vi "THzTime_SPEED_control_reduced.vi"(1 "ESP300 Axis":i8=1, 2 "ESP300 Address":string="1", 4 "Lockin Address":string="12") -> ()   [LabVIEW 2010]
panel:
  in  "Axis Number":u8
  in  "SHOT202 Address":string
  in  "reference postion":dbl
  in  "sample position":dbl
  in  "number of measurement":dbl
  in  "Interdelay (ms)":dbl
  in  "pre delay(ms)":dbl=10.0
  in  "Reset Range":bool
  out "Lock-in Y-Channel":dbl=2.5466e-11 format="%#.3p"
  out "Lock-in X-Channel":dbl=-5.457e-12 format="%#.3p"
  out "THz Time-domain Signal Wave":cluster{"x-axis":sgl[], "y-axis":dbl[]}(graph)={"x-axis"=[-3.0, -2.99, -2.98, -2.97, -2.96, -2.95, -2.94, -2.93, -2.92, -2.91, -2.9, -2.89, -2.88, -2.87, -2.86, -2.85, -2.84, -2.83, -2.82, -2.81, -2.8, -2.79, -2.78, -2.77, -2.76, -2.75, -2.74, -2.73, -2.72, -2.71, -2.7, -2.69, -2.68, -2.67, -2.66, -2.65, -2.64, -2.63, -2.6200001, -2.61, -2.6, -2.59, -2.58, -2.57, -2.56, -2.55, -2.54, -2.53, -2.52, -2.51, -2.5, -2.49, -2.48, -2.47, -2.46, -2.45, -2.44, -2.43, -2.42, -2.41, -2.4, -2.39, -2.38, -2.3700001, -2.3600001, -2.35, -2.34, -2.33, -2.32, -2.31, -2.3, -2.29, -2.28, -2.27, -2.26, -2.25, -2.24, -2.23, -2.22, -2.21, -2.2, -2.19, -2.18, -2.17, -2.16, -2.15, -2.14, -2.13, -2.1200001, -2.1100001, -2.1, -2.09, -2.08, -2.07, -2.06, -2.05, -2.04, -2.03, -2.02, -2.01, -2.0, -1.99, -1.98, -1.97, -1.96, -1.95, -1.94, -1.9300001, -1.9200001, -1.91, -1.9, -1.89, -1.88, -1.87, -1.86, -1.85, -1.84, -1.83, -1.82, -1.8100001, -1.8000001, -1.7900001, -1.78, -1.77, -1.76, -1.75, -1.74, -1.73, -1.72, -1.71, -1.7, -1.69, -1.6800001, -1.6700001, -1.6600001, -1.65, -1.64, -1.63, -1.62, -1.61, -1.6, -1.59, -1.58, -1.57, -1.5600001, -1.5500001, -1.5400001, -1.5300001, -1.52, -1.51, -1.5, -1.49, -1.48, -1.47, -1.46, -1.45, -1.44, -1.4300001, -1.4200001, -1.4100001, -1.4000001, -1.39, -1.38, -1.37, -1.36, -1.35, -1.34, -1.33, -1.32, -1.3100001, -1.3000001, -1.2900001, -1.2800001, -1.27, -1.26, -1.25, -1.24, -1.23, -1.22, -1.21, -1.2, -1.19, -1.1800001, -1.1700001, -1.1600001, -1.1500001, -1.14, -1.13, -1.12, -1.11, -1.1, -1.09, -1.08, -1.07, -1.0600001, -1.0500001, -1.0400001, -1.0300001, -1.0200001, -1.01, -1.0, -0.99000007], "y-axis"=[6.18461e-11, 6.18461e-11, 6.275559999999999e-11, 6.457460000000001e-11, 6.54841e-11, 6.63936e-11, 6.821255e-11, 7.00315e-11, 7.18505e-11, 7.36695e-11, 7.54885e-11, 7.6398e-11, 7.6398e-11, 7.8217e-11, 7.8217e-11, 7.8217e-11, 7.8217e-11, 7.8217e-11, 7.8217e-11, 7.8217e-11, 7.8217e-11, 7.8217e-11, 7.8217e-11, 7.8217e-11, 7.73075e-11, 7.6398e-11, 7.54885e-11, 7.4579e-11, 7.4579e-11, 7.4579e-11, 7.4579e-11, 7.4579e-11, 7.4579e-11, 7.4579e-11, 7.36695e-11, 7.276e-11, 7.276e-11, 7.276e-11, 7.18505e-11, 7.18505e-11, 7.276e-11, 7.18505e-11, 7.0941e-11, 7.0941e-11, 7.00315e-11, 6.9122e-11, 6.821255e-11, 6.63936e-11, 6.457460000000001e-11, 6.275559999999999e-11, 6.18461e-11, 6.18461e-11, 6.275559999999999e-11, 6.36651e-11, 6.63936e-11, 6.912205e-11, 7.275999999999999e-11, 7.6398e-11, 7.91265e-11, 8.09455e-11, 8.27645e-11, 8.3674e-11, 8.3674e-11, 8.3674e-11, 8.27645e-11, 8.09455e-11, 7.821699999999999e-11, 7.36695e-11, 6.821255e-11, 6.09366e-11, 5.54795e-11, 4.911295e-11, 4.2746500000000003e-11, 3.7289500000000003e-11, 3.2742e-11, 3.001355e-11, 2.7285e-11, 2.7285e-11, 2.819455e-11, 3.092305e-11, 3.4561000000000003e-11, 3.7289500000000003e-11, 3.9108499999999995e-11, 4.09275e-11, 4.45655e-11, 4.638445e-11, 5.00224e-11, 5.18414e-11, 5.36604e-11, 5.72985e-11, 5.82081e-11, 5.82081e-11, 5.82081e-11, 6.00271e-11, 6.09366e-11, 6.275559999999999e-11, 6.457460000000001e-11, 6.730305e-11, 7.00315e-11, 7.18505e-11, 7.36695e-11, 7.54885e-11, 7.6398e-11, 7.73075e-11, 7.8217e-11, 7.8217e-11, 7.8217e-11, 7.8217e-11, 7.8217e-11, 7.8217e-11, 7.8217e-11, 7.8217e-11, 7.8217e-11, 7.8217e-11, 7.8217e-11, 7.8217e-11, 7.91265e-11, 8.0036e-11, 8.0036e-11, 7.91265e-11, 7.8217e-11, 7.8217e-11, 7.8217e-11, 7.8217e-11, 7.91265e-11, 8.0036e-11, 8.0036e-11, 8.0036e-11, 8.09455e-11, 8.1855e-11, 8.09455e-11, 8.0036e-11, 7.91265e-11, 7.8217e-11, 7.8217e-11, 7.73075e-11, 7.54885e-11, 7.36695e-11, 7.18505e-11, 6.9122e-11, 6.73031e-11, 6.54841e-11, 6.457460000000001e-11, 6.36651e-11, 6.275559999999999e-11, 6.09366e-11, 6.00271e-11, 6.00271e-11, 6.00271e-11, 6.00271e-11, 6.09366e-11, 6.18461e-11, 6.18461e-11, 6.18461e-11, 6.275559999999999e-11, 6.36651e-11, 6.457460000000001e-11, 6.54841e-11, 6.457460000000001e-11, 6.36651e-11, 6.36651e-11, 6.36651e-11, 6.36651e-11, 6.36651e-11, 6.36651e-11, 6.36651e-11, 6.36651e-11, 6.36651e-11, 6.36651e-11, 6.36651e-11, 6.36651e-11, 6.36651e-11, 6.457460000000001e-11, 6.54841e-11, 6.457460000000001e-11, 6.457460000000001e-11, 6.54841e-11, 6.63936e-11, 6.73031e-11, 6.73031e-11, 6.9122e-11, 6.73031e-11, 6.821255e-11, 6.9122e-11, 6.9122e-11, 6.73031e-11, 6.821255e-11, 6.9122e-11, 6.9122e-11, 6.9122e-11, 6.9122e-11, 6.821255e-11, 6.73031e-11, 6.73031e-11, 6.73031e-11, 6.73031e-11, 6.73031e-11, 6.73031e-11, 6.63936e-11, 6.63936e-11, 6.54841e-11, 6.54841e-11]}
  in  "Autosave Directory for Long-term Average Scan":path=path "D:/KHA/20140828_reference/20140829/MAX1"
  in  "OK Button":bool
  out "Data Type":string="outp ? 1"
  in  "Enum":enum16{"X", "Y", "Abs"}(ring)
  in  "Draw":bool
  in  "Exit Program":bool
  in  "Short term \nAverage#":i8=2
  in  "Step":sgl=0.01 min=0 max=10000 format="%.3f"
  in  "End Position":sgl=-1.0 min=-75 max=75 format="%#.3f"
  in  "Start Position":sgl=-3.0 min=-75 max=75 format="%#.3f"
  # "This Program Run First (1) and then Run the Approach Program (2)"
  # "THz Experiment"
  # "Data"
  # "Auto-offset"
  # "Start Position (mm)"
  # "End Position (mm)"
  # "Step (mm)"
  # "Point Avg"
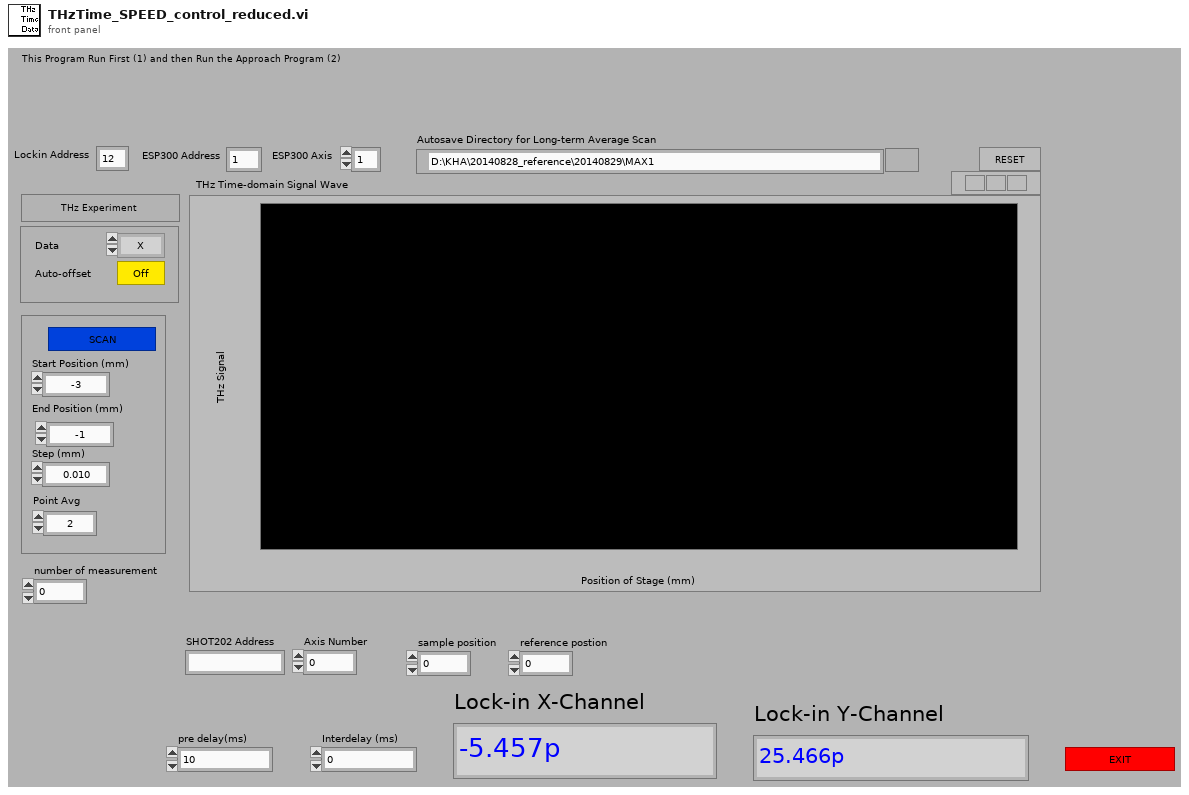
[diagram p1: front panel]
types:
  T1 = cluster{"Step Number":i32, "Step":sgl, "Start Position":sgl, "Time-out":i32, "Lockin Address":string, "Short term \nAverage#":i8, i32, "ESP300 Axis":i8, "Value":string, "pre delay(ms)":dbl, "Interdelay (ms)":dbl, "Autosave Directory for Long-term Average Scan":path}
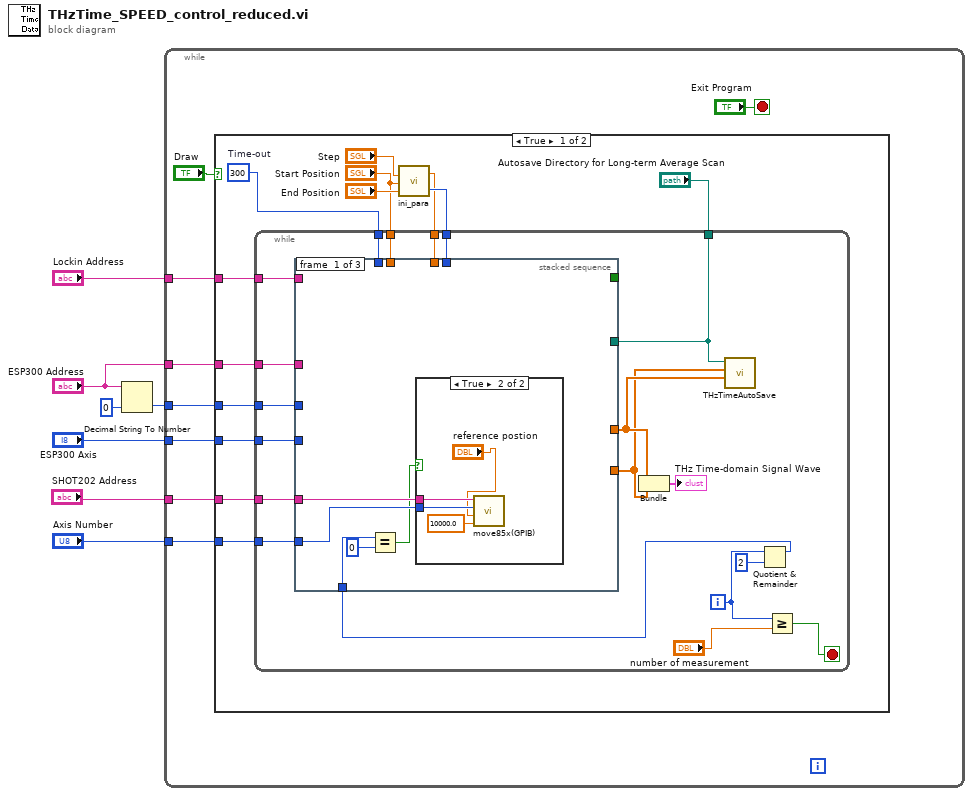
[diagram p0: block diagram]
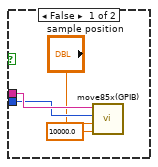
[diagram p2: hidden frame]
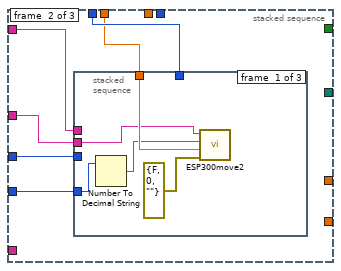
[diagram p3: hidden frame]
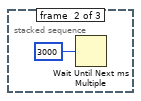
[diagram p4: hidden frame]
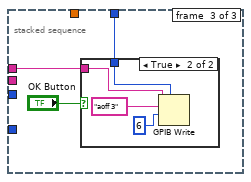
[diagram p5: hidden frame]
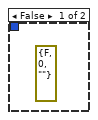
[diagram p6: hidden frame]
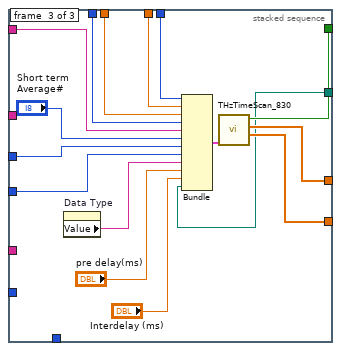
[diagram p7: hidden frame]
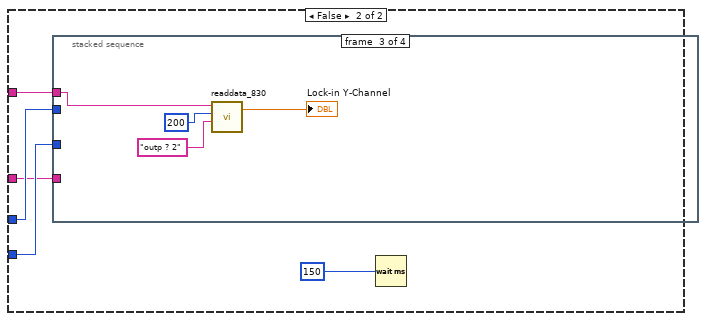
[diagram p8: hidden frame]
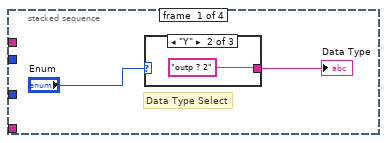
[diagram p9: hidden frame]
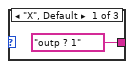
[diagram p10: hidden frame]
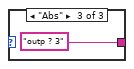
[diagram p11: hidden frame]
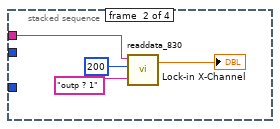
[diagram p12: hidden frame]
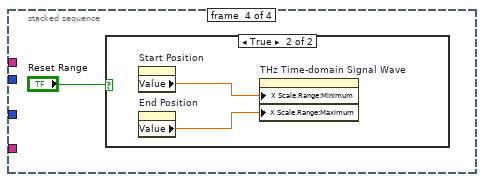
[diagram p13: hidden frame]
diagram:
  n1 = Decimal String To Number(string="ESP300 Address", default (0L)=0 ("default (0 I32)")) -> (number=w5:i32)  [unwired: 1 in, 1 out]
  n2 = while {
    tunnel: "ESP300 Axis" -> [w13]
    tunnel: "Lockin Address" -> [w12]
    tunnel: w5 -> [w11]
    tunnel: "ESP300 Address" -> [w10]
    tunnel: "SHOT202 Address" -> [w9]
    tunnel: "Axis Number" -> [w8]
    stop <- "Exit Program" stop-if-true
    n3 = case shown="True" "Draw" {
      tunnel: w12 -> [w28 w98]
      tunnel: w13 -> [w27 w100]
      tunnel: w11 -> [w26 w99]
      tunnel: w10 -> [w18 w96]
      tunnel: w9 -> [w17 _]
      tunnel: w8 -> [w16 _]
      frame True {
        w25 = 300  # Time-out
        n4 = call "ini_para.vi"("End Position"="End Position", "Start Position"="Start Position", "Step"="Step") -> ("Step Number"=w22:i32, "Step"=w21:sgl)
        n5 = while {
          tunnel: w28 -> [w47]
          tunnel: w27 -> [w46]
          tunnel: w26 -> [w45]
          tunnel: w25 -> [w44]
          tunnel: w22 -> [w43]
          tunnel: w21 -> [w42]
          tunnel: "Start Position" -> [w41]
          tunnel: "Autosave Directory for Long-term Average Scan" -> [w40]
          tunnel: w18 -> [w39]
          tunnel: w17 -> [w33]
          tunnel: w16 -> [w32]
          i -> [w31]
          stop <- w34 stop-if-true
          n6 = Quotient & Remainder(x=w31, y=2) -> (x-y*floor(x/y)=w29:i32)  [unwired: 1 out]
          n7 = stacked-sequence {
            tunnel: w47 -> [_ w66 w91]
            tunnel: w44 -> [_ w65 w92]
            tunnel: [_ _ w86] -> _
            tunnel: w46 -> [_ w64 w88]
            tunnel: w45 -> [_ w63 w89]
            tunnel: w41 -> [_ w62 w93]
            tunnel: w42 -> [_ _ w94]
            tunnel: w43 -> [_ _ w95]
            tunnel: [_ _ w85] -> w38
            tunnel: [_ _ w84] -> w36
            tunnel: w39 -> [_ w61 _]
            tunnel: w40 -> [_ _ w80]
            tunnel: w33 -> [w52 _ _]
            tunnel: w32 -> [w51 _ _]
            tunnel: w29 -> [w50 _ _]
            frame #0 {
              n8 = Equal?(x=w50, y=0) -> (x = y?=w48:bool)
              n9 = case shown="True" w48 {
                tunnel: w52 -> [w56 w60]
                tunnel: w51 -> [w55 w59]
                frame False {
                  n10 = call "move85x(GPIB).vi"("wait time(ms)"=10000.0, "Moving Distance (mm) : resolutino is 1um"="sample position", "Axis Number"=w55, "SHOT202 Address"=w56) -> ()
                }
                frame True {
                  n11 = call "move85x(GPIB).vi"("wait time(ms)"=10000.0, "Moving Distance (mm) : resolutino is 1um"="reference postion", "Axis Number"=w59, "SHOT202 Address"=w60) -> ()
                }
              }
            }
            frame #1 {
              n12 = stacked-sequence {
                tunnel: w66 -> [_ _ w74]
                tunnel: w65 -> [_ _ w73]
                tunnel: w64 -> [w68 _ _]
                tunnel: w63 -> [_ _ _]
                tunnel: w62 -> [w71 _ _]
                tunnel: w61 -> [w69 _ _]
                frame #0 {
                  n13 = Number To Decimal String(number=w68) -> (decimal integer string=w67:string)  [unwired: 1 in]
                  n14 = call "ESP300move2.vi"("ESP300 Address"=w69, "ESP300 Channel"=w67, "Target"=w71, "error in (no error) 2"=errorcluster {"status"=FALSE, "code"=0, "source"=""}) -> ()  [unwired: 6 in, 1 out]
                }
                frame #1 {
                  n15 = Wait Until Next ms Multiple(millisecond multiple=3000) -> ()  [unwired: 1 out]
                }
                frame #2 {
                  n16 = case shown="True" "OK Button" {
                    tunnel: w74 -> [_ w79]
                    tunnel: w73 -> [_ w77]
                    frame False {
                      (unwired) errorcluster {"status"=FALSE, "code"=0, "source"=""} ("error in")
                    }
                    frame True {
                      n17 = GPIB Write(0:w79, 1:"aoff 3" ("data"), 2:i16 6 ("mode (0)"), 4:w77) -> ()  [unwired: 1 in, 2 out]
                    }
                  }
                }
              }
            }
            frame #2 {
              n18 = property on="Data Type" class="Str"() -> ("Value"=w87:string)  [unwired: 2 in, 2 out]
              n19 = Bundle("Step Number"=w95, "Step"=w94, "Start Position"=w93, "Time-out"=w92, "Lockin Address"=w91, "Short term \nAverage#"="Short term \nAverage#", w89, "ESP300 Axis"=w88, "Value"=w87, "pre delay(ms)"="pre delay(ms)", "Interdelay (ms)"="Interdelay (ms)", "Autosave Directory for Long-term Average Scan"=w80) -> (w83:T1)  [unwired: 1 in]
              n20 = call "THzTimeScan_830.vi"("input"=w83) -> ("loop stop"=w86:bool, "x-axis"=w85:sgl[], "y-axis"=w84:dbl[])  [unwired: 1 in]
            }
          }
          n21 = Bundle("x-axis"=w38, "y-axis"=w36) -> (→"THz Time-domain Signal Wave":cluster{"x-axis":sgl[], "y-axis":dbl[]})  [unwired: 1 in]
          n22 = call "THzTimeAutoSave.vi"("x-axis"=w38, "y-axis"=w36, "Autosave Directory for Long-term Average Scan"=w40) -> ()  [unwired: 1 in]
          n23 = Greater Or Equal?(x=w31, y="number of measurement") -> (x >= y?=w34:bool)
        }
      }
      frame False {
        n24 = stacked-sequence {
          tunnel: w100 -> [_ _ _ _]
          tunnel: w99 -> [_ _ _ _]
          tunnel: w98 -> [_ w109 w113 _]
          tunnel: w96 -> [_ _ _ _]
          frame #0 {
            # "Data Type Select"
            n25 = case shown="\"Y\"" "Enum" {
              tunnel: ["outp ? 1" "outp ? 2" "outp ? 3"] -> w102
              frame "X", Default {
              }
              frame "Y" {
              }
              frame "Abs" {
              }
            }
            "Data Type" <- w102
          }
          frame #1 {
            n26 = call "readdata_830.vi"("Command"="outp ? 1", "timeout"=200, "Lockin Address"=w109) -> ("Data"=→"Lock-in X-Channel":dbl)  [unwired: 1 in, 1 out]
          }
          frame #2 {
            n27 = call "readdata_830.vi"("Command"="outp ? 2", "timeout"=200, "Lockin Address"=w113) -> ("Data"=→"Lock-in Y-Channel":dbl)  [unwired: 1 in, 1 out]
          }
          frame #3 {
            n28 = case shown="True" "Reset Range" {
              frame False {
              }
              frame True {
                n29 = property on="Start Position" class="DigNum (strict)"() -> ("Value"=w116:sgl)  [unwired: 2 in, 2 out]
                n30 = property on="End Position" class="DigNum (strict)"() -> ("Value"=w115:sgl)  [unwired: 2 in, 2 out]
                n31 = property on="THz Time-domain Signal Wave" class="XYGraph (strict)"("X Scale.Range:Minimum"=w116, "X Scale.Range:Maximum"=w115) -> ()  [unwired: 2 in, 2 out]
              }
            }
          }
        }
        n32 = Wait (ms)(milliseconds to wait=u32 150) -> ()  [unwired: 1 out]
      }
    }
  }
